vi "Do.vi"(8 "error in (no error)":errorcluster, 9 "Events":refnum<class "Events.lvclass">, 10 "Message Loop Data in":T1, 11 "IUnregister in":refnum<class "IUnregister.lvclass">) -> (0 "error out":errorcluster, 1 "Write request":T9, 2 "Message Loop Data out":T1, 3 "IUnregister out":refnum<class "IUnregister.lvclass">)   [LabVIEW 2020, in "wamplv.lvlib" / "IUnregister.lvclass"]
uses:
  IUnregister.lvclass
  WAMP Client/WAMP Client.lvclass
  WAMP Client/Private/TypeDef/Publish Requests Map.ctl
  wamplv.lvlib
  WAMP Client/Private/TypeDef/Endpoint Data.ctl
  Call/ICallRequest/ICallRequest.lvclass
  WAMP Client/Private/TypeDef/CALL Request Map.ctl
  WAMP Client/Private/TypeDef/SUBSCRIBE Requests Map.ctl
  WAMP Client/Private/TypeDef/Subscriptions Map.ctl
  WAMP Client/Private/TypeDef/Unsubscribe Requests Map.ctl
  WAMP Client/Private/TypeDef/Unregister requests map.ctl
  WAMP Client/Private/TypeDef/Message Loop Data.ctl
  TypeDefs/Transport type.ctl
  WAMP Client/Private/TypeDef/Write queue item.ctl
  Events/EventsParent/Events.lvclass
  Subscribe/ISubscribe/ISubscribe.lvclass
  Publish/IPublish/IPublish.lvclass
  Message loop classes/Subscription details/SubscriptionDetailsParent/SubscriptionDetailsParent.lvclass
  Unsubscribe/IUnsubscribe/IUnsubscribe.lvclass
  Register/IRegister/IRegister.lvclass
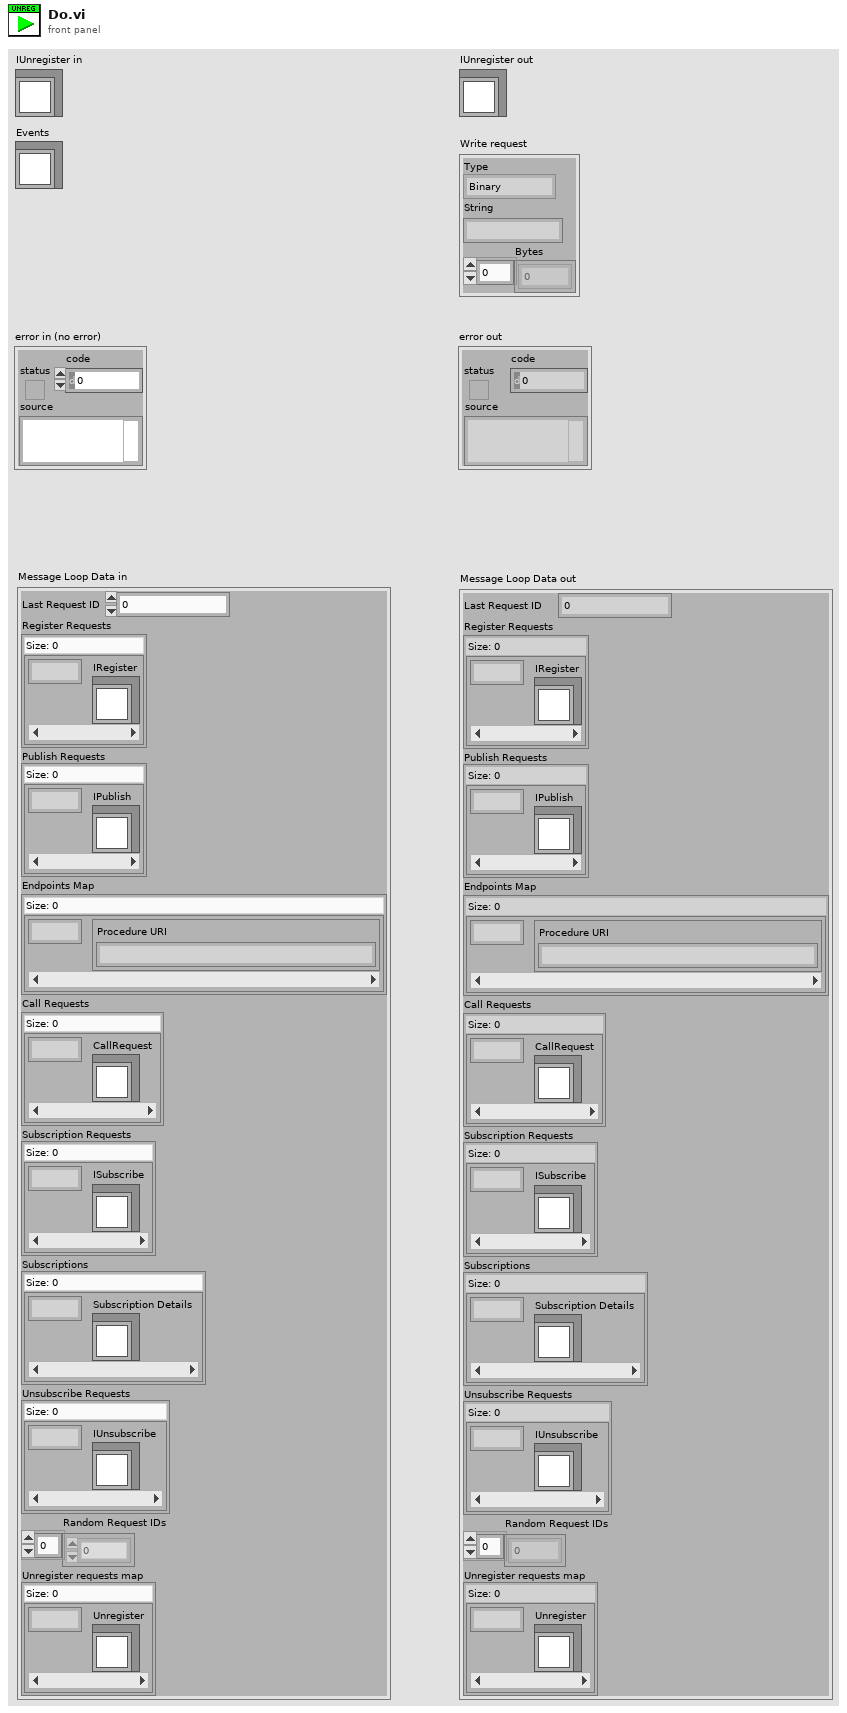
[diagram p1: front panel]
types:
  T1 = typedef "wamplv.lvlib/Message Loop Data.ctl" = cluster{"Last Request ID":u64, "Register Requests":map{u64, refnum<class "IRegister.lvclass">}, "Publish Requests":T2, "Endpoints Map":map{u64, T3}, "Call Requests":T4, "Subscription Requests":T5, "Subscriptions":T6, "Unsubscribe Requests":T7, "Random Request IDs":u64[], "Unregister requests map":T8}
  T2 = typedef "wamplv.lvlib/Publish Requests Map.ctl" = map{u64, refnum<class "IPublish.lvclass">}
  T3 = typedef "wamplv.lvlib/Endpoint Data.ctl" = cluster{"Procedure URI":string}
  T4 = typedef "wamplv.lvlib/CALL Request Map.ctl" = map{u64, refnum<class "ICallRequest.lvclass">}
  T5 = typedef "wamplv.lvlib/SUBSCRIBE Requests Map.ctl" = map{u64, refnum<class "ISubscribe.lvclass">}
  T6 = typedef "wamplv.lvlib/Subscriptions Map.ctl" = map{u64, refnum<class "SubscriptionDetailsParent.lvclass">}
  T7 = typedef "wamplv.lvlib/Unsubscribe Requests Map.ctl" = map{u64, refnum<class "IUnsubscribe.lvclass">}
  T8 = typedef "wamplv.lvlib/Unregister requests map.ctl" = map{u64, refnum<class "IUnregister.lvclass">}
  T9 = typedef "wamplv.lvlib/Write queue item.ctl" = cluster{"Type":T10, "String":string, "Bytes":u8[]}
  T10 = typedef "wamplv.lvlib/Transport type.ctl" = enum16{"Binary", "Text"}
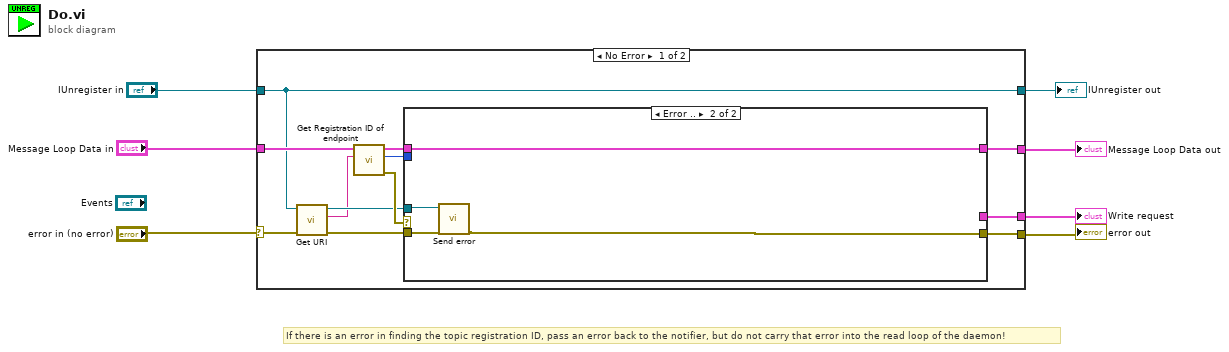
[diagram p0: block diagram]
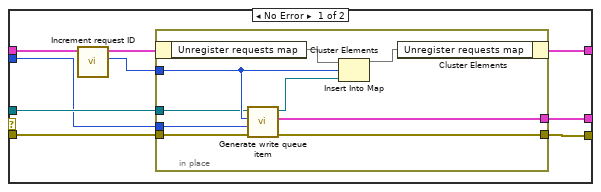
[diagram p2: hidden frame]
diagram:
  # "If there is an error in finding the topic registration ID, pass an error back to the notifier, but do not carry that error into the read loop of the daemon!"
  n1 = case shown="No Error" "error in (no error)" {
    selector: "error in (no error)" -> [w12 w43]
    tunnel: [w18 w43] -> w7
    tunnel: "Message Loop Data in" -> [w17 w42]
    tunnel: [w13 w42] -> w5
    tunnel: [w11 _] -> w3
    tunnel: "IUnregister in" -> [w8 w41]
    tunnel: [w8 w41] -> w1
    frame No Error {
      n2 = call-dynamic "Get URI.vi"("IUnregister in"=w8) -> ("URL"=w9:string, "IUnregister out"=w10:refnum<class "IUnregister.lvclass">)  [unwired: 9 in]
      n3 = call "Get Registration ID of endpoint.vi"("Endpoint URI"=w9, "Message loop data (in)"=w17) -> ("error out"=w14:errorcluster, "Registrtion ID"=w15:u64, "Message loop data (out)"=w16:T1)  [unwired: 7 in]
      n4 = case shown="Error .." w14 {
        tunnel: [w20 w37] -> w18
        tunnel: w10 -> [w27 w38]
        tunnel: w16 -> [w26 w40]
        tunnel: w15 -> [w21 _]
        tunnel: [w24 w40] -> w13
        tunnel: w12 -> [w22 w39]
        tunnel: [w19 _] -> w11
        frame No Error {
          n5 = call "Increment request ID.vi"("Message Loop Shift Register Data (in)"=w26) -> ("New Request ID"=w23:u64, "Message Loop Shift Register Data (out)"=w25:T1)  [unwired: 9 in]
          n6 = in-place "In Place Element Structure" {
            in-place-border: w27 -> [w31]
            in-place-border: w23 -> [w32]
            in-place-border: w22 -> [w34]
            in-place-border: w21 -> [w33]
            in-place-border: [w29] -> w20
            in-place-border: [w28] -> w19
            n7 = in-place-cluster #1(w25) -> ("Unregister requests map"=w36:T8)
            n8 = call-dynamic "Generate write queue item.vi"("error in (no error)"=w34, "Registration ID"=w33, "Request ID"=w32, "IUnregister in"=w31) -> ("error out"=w29:errorcluster, "Write queue item"=w28:T9, "IUnregister out"=w30:refnum<class "IUnregister.lvclass">)  [unwired: 5 in]
            n9 = Insert Into Map(map in=w36, key=w32, value=w30) -> (map out=w35:T8)  [unwired: 2 out]
            n10 = in-place-cluster #1("Unregister requests map"=w35) -> (w24:T1)
          }
        }
        frame Error {
          n11 = call-dynamic "Send error.vi"("error in (no error)"=w39, "IUnregister in"=w38) -> ("error out"=w37:errorcluster)  [unwired: 8 in, 1 out]
        }
      }
    }
    frame Error {
    }
  }
  "error out" <- w7
  "IUnregister out" <- w1
  "Write request" <- w3
  "Message Loop Data out" <- w5
